vi "telemetria.vi"(11 "Output Array":string[][](array[string])) -> (0 "v3":u16, 1 "sr v2":dbl format="%0.2f", 2 "v2":u16, 3 "œr v1":dbl format="%0.2f", 4 "sr v3":dbl format="%0.2f", 5 "v 1":u16, 6 "œrednie":T1, 8 "raw":cluster{u16, u16, u16, u16, u16, u16})   [LabVIEW 2015]
uses:
  <vilib>/ptbypt/NI_PtbyPt.lvlib
panel:
  out "Result":string
  out "match + rest of string":string
  out "substring before match":string
  out "concatenated string":string
  out "element 3":string
  out "œr v1  2":dbl format="%0.2f"
  out "sr v2 2":dbl format="%0.2f"
  out "v 2":u16
  out "v2 2":u16
  out "sr v3 2":dbl format="%0.2f"
  out "v3  2":u16
  out "element 2":string
  out "element":string
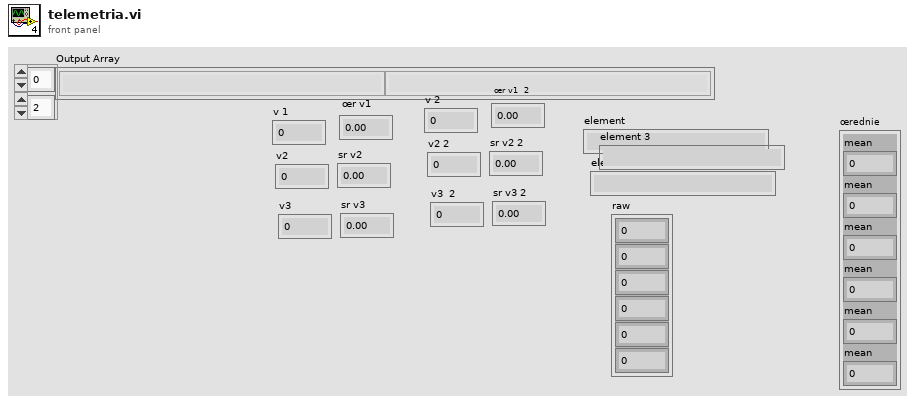
[diagram p1: front panel]
types:
  T1 = cluster{"mean":dbl, "mean":dbl, "mean":dbl, "mean":dbl, "mean":dbl, "mean":dbl}
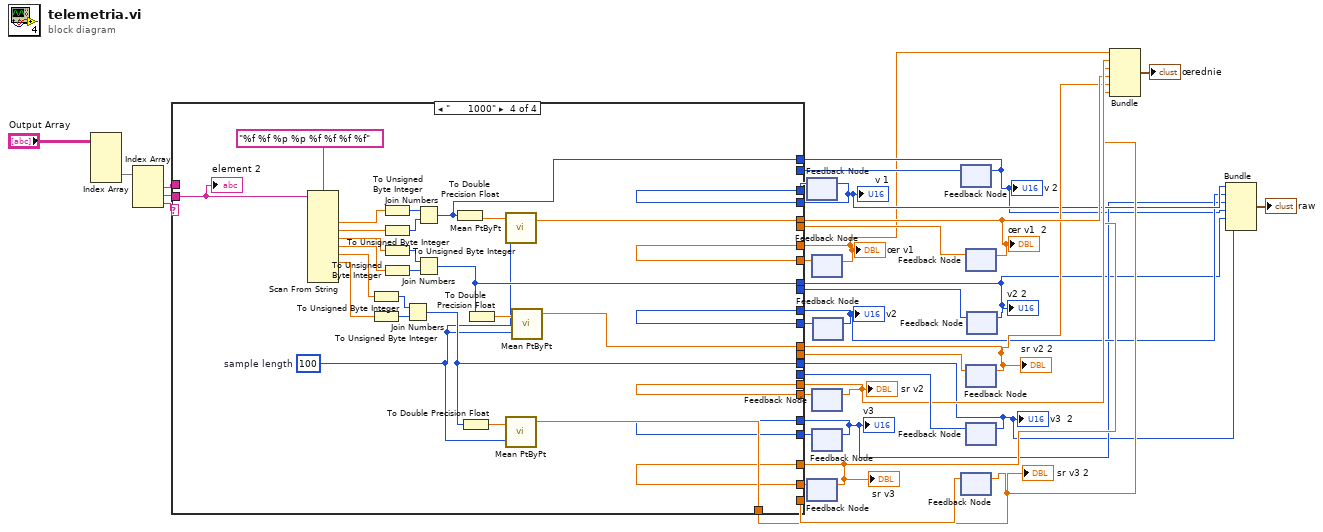
[diagram p0: block diagram]
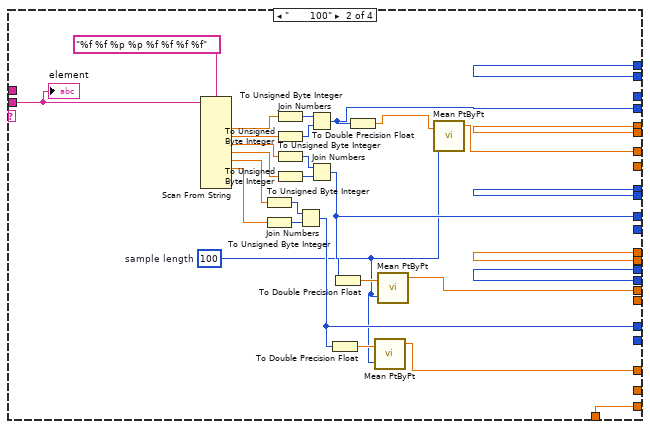
[diagram p3: hidden frame]
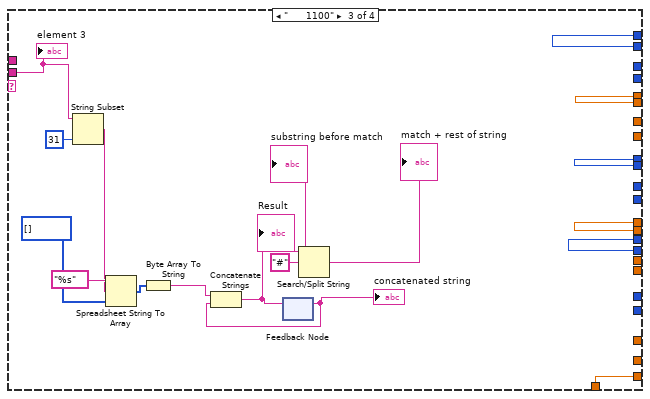
[diagram p4: hidden frame]
diagram:
  n1 = Index Array(array="Output Array") -> (element #2=w30:string[])  [unwired: 4 in, 1 out]
  n2 = Index Array(array=w30) -> (element #1=w23:string, element #2=w29:string, element #3=w28:string)  [unwired: 3 in]
  n3 = feedback #1() -> (w25:u16)  [unwired: 1 in]
  n4 = feedback #2() -> (w21:dbl)  [unwired: 1 in]
  n5 = feedback #3() -> (w26:dbl)  [unwired: 1 in]
  n6 = feedback #4() -> (w27:dbl)  [unwired: 1 in]
  n7 = feedback #5() -> (w22:u16)  [unwired: 1 in]
  n8 = feedback #6() -> (w24:u16)  [unwired: 1 in]
  n9 = feedback #7() -> (w20:u16)  [unwired: 1 in]
  n10 = feedback #8() -> (w15:dbl)  [unwired: 1 in]
  n11 = feedback #9() -> (w19:dbl)  [unwired: 1 in]
  n12 = feedback #10() -> (w17:dbl)  [unwired: 1 in]
  n13 = feedback #11() -> (w16:u16)  [unwired: 1 in]
  n14 = feedback #12() -> (w18:u16)  [unwired: 1 in]
  n15 = case shown="\"      1000\"" w28 {
    tunnel: w29 -> [_ w64 w83 w112]
    tunnel: [w42 w63 _ w98] -> w1
    tunnel: [w43 w62 _ w96] -> w14
    tunnel: w27 -> [w43 _ _ w96]
    tunnel: w26 -> [w42 _ _ w98]
    tunnel: [w41 w51 _ w99] -> w8
    tunnel: [w40 w61 _ w97] -> w7
    tunnel: w25 -> [w41 _ _ w99]
    tunnel: w24 -> [w40 _ _ w97]
    tunnel: w23 -> [_ _ _ _]
    tunnel: [w39 w54 _ w95] -> w6
    tunnel: [w38 w53 _ w94] -> w13
    tunnel: w22 -> [w39 _ _ w95]
    tunnel: w21 -> [w38 _ _ w94]
    tunnel: [w37 w50 w91 w104] -> w5
    tunnel: [w36 w49 w90 w92] -> w12
    tunnel: [w35 w48 w89 w103] -> w4
    tunnel: [w34 w47 w88 w102] -> w11
    tunnel: [w33 w46 w87 w101] -> w3
    tunnel: [w32 w45 w86 w100] -> w10
    tunnel: w20 -> [w37 w50 w91 _]
    tunnel: w19 -> [w36 w49 w90 _]
    tunnel: w18 -> [w35 w48 w89 _]
    tunnel: w17 -> [w34 w47 w88 _]
    tunnel: w16 -> [w33 w46 w87 _]
    tunnel: w15 -> [w32 w45 w86 _]
    frame "False", Default {
    }
    frame "       100" {
      w44 = 100  # sample length
      n16 = Scan From String(format string="%f %f %p %p %f %f %f %f", input string=w64) -> (output 1=w72:dbl, output 2=w71:dbl, output 3=w70:dbl, output 4=w67:dbl, output 5=w57:dbl, output 6=w56:dbl)  [unwired: 12 in, 3 out]
      n17 = To Unsigned Byte Integer(number=w57) -> (unsigned 8bit integer=w58:u8)
      n18 = To Unsigned Byte Integer(number=w56) -> (unsigned 8bit integer=w59:u8)
      n19 = To Unsigned Byte Integer(number=w72) -> (unsigned 8bit integer=w69:u8)
      n20 = To Unsigned Byte Integer(number=w71) -> (unsigned 8bit integer=w68:u8)
      n21 = To Unsigned Byte Integer(number=w70) -> (unsigned 8bit integer=w66:u8)
      n22 = To Unsigned Byte Integer(number=w67) -> (unsigned 8bit integer=w65:u8)
      n23 = Join Numbers(hi=w58, lo=w59) -> ((hi.lo)=w54:u16)
      n24 = Join Numbers(hi=w69, lo=w68) -> ((hi.lo)=w51:u16)
      n25 = Join Numbers(hi=w66, lo=w65) -> ((hi.lo)=w61:u16)
      n26 = To Double Precision Float(number=w54) -> (double precision float=w55:dbl)
      n27 = To Double Precision Float(number=w61) -> (double precision float=w60:dbl)
      n28 = To Double Precision Float(number=w51) -> (double precision float=w52:dbl)
      n29 = call <vilib>:"Mean PtByPt.vi"("x"=w55, "sample length"=w44) -> ("mean"=w53:dbl)  [unwired: 2 in, 1 out]
      n30 = call <vilib>:"Mean PtByPt.vi"("x"=w60, "sample length"=w44) -> ("mean"=w62:dbl)  [unwired: 2 in, 1 out]
      n31 = call <vilib>:"Mean PtByPt.vi"("x"=w52, "sample length"=w44) -> ("mean"=w63:dbl)  [unwired: 2 in, 1 out]
      "element" <- w64
    }
    frame "      1100" {
      n32 = String Subset(string=w83, length (rest)=31 ("length (rest)")) -> (substring=w81:string)  [unwired: 1 in]
      n33 = Spreadsheet String To Array(format string="%s", spreadsheet string=w81, array type (2D Dbl)=u8[] [] ("unsigned byte array")) -> (array=w80:u8[])  [unwired: 1 in]
      n34 = Byte Array To String(unsigned byte array=w80) -> (string=w74:string)
      n35 = feedback #13() -> (w79:string)  [unwired: 1 in]
      "concatenated string" <- w79
      n36 = Concatenate Strings(w74, w79) -> (w78:string)
      n37 = feedback-in #13(w78) -> ()
      n38 = Search/Split String(string=w78, search string/char (-)="#") -> (substring before match=→"substring before match":string, match + rest of string=→"match + rest of string":string)  [unwired: 1 in, 1 out]
      "element 3" <- w83
    }
    frame "      1000" {
      w93 = 100  # sample length
      n39 = Scan From String(format string="%f %f %p %p %f %f %f %f", input string=w112) -> (output 1=w120:dbl, output 2=w119:dbl, output 3=w118:dbl, output 4=w115:dbl, output 5=w108:dbl, output 6=w107:dbl)  [unwired: 12 in, 3 out]
      n40 = To Unsigned Byte Integer(number=w108) -> (unsigned 8bit integer=w109:u8)
      n41 = To Unsigned Byte Integer(number=w107) -> (unsigned 8bit integer=w110:u8)
      n42 = To Unsigned Byte Integer(number=w120) -> (unsigned 8bit integer=w117:u8)
      n43 = To Unsigned Byte Integer(number=w119) -> (unsigned 8bit integer=w116:u8)
      n44 = To Unsigned Byte Integer(number=w118) -> (unsigned 8bit integer=w114:u8)
      n45 = To Unsigned Byte Integer(number=w115) -> (unsigned 8bit integer=w113:u8)
      n46 = Join Numbers(hi=w109, lo=w110) -> ((hi.lo)=w101:u16)
      n47 = Join Numbers(hi=w117, lo=w116) -> ((hi.lo)=w104:u16)
      n48 = Join Numbers(hi=w114, lo=w113) -> ((hi.lo)=w103:u16)
      n49 = To Double Precision Float(number=w104) -> (double precision float=w105:dbl)
      n50 = To Double Precision Float(number=w101) -> (double precision float=w106:dbl)
      n51 = To Double Precision Float(number=w103) -> (double precision float=w111:dbl)
      n52 = call <vilib>:"Mean PtByPt.vi"("x"=w105, "sample length"=w93) -> ("mean"=w92:dbl)  [unwired: 2 in, 1 out]
      n53 = call <vilib>:"Mean PtByPt.vi"("x"=w106, "sample length"=w93) -> ("mean"=w100:dbl)  [unwired: 2 in, 1 out]
      n54 = call <vilib>:"Mean PtByPt.vi"("x"=w111, "sample length"=w93) -> ("mean"=w102:dbl)  [unwired: 2 in, 1 out]
      "element 2" <- w112
    }
  }
  "œr v1" <- w1
  "sr v2" <- w14
  "v 1" <- w8
  "v2" <- w7
  "sr v3" <- w13
  "v3" <- w6
  "œr v1  2" <- w12
  "sr v2 2" <- w11
  "v 2" <- w5
  "v2 2" <- w4
  "sr v3 2" <- w10
  "v3  2" <- w3
  n55 = feedback-in #1(w8) -> ()
  n56 = feedback-in #2(w13) -> ()
  n57 = feedback-in #3(w1) -> ()
  n58 = feedback-in #4(w14) -> ()
  n59 = feedback-in #5(w6) -> ()
  n60 = feedback-in #6(w7) -> ()
  n61 = feedback-in #7(w5) -> ()
  n62 = feedback-in #8(w10) -> ()
  n63 = feedback-in #9(w12) -> ()
  n64 = feedback-in #10(w11) -> ()
  n65 = feedback-in #11(w3) -> ()
  n66 = feedback-in #12(w4) -> ()
  n67 = Bundle("mean"=w1, "mean"=w14, "mean"=w13, "mean"=w12, "mean"=w11, "mean"=w10) -> (→"œrednie":T1)  [unwired: 1 in]
  n68 = Bundle(w8, w7, w6, w5, w4, w3) -> (→"raw":cluster{u16, u16, u16, u16, u16, u16})  [unwired: 1 in]
